vi "send.vi"() -> ()   [LabVIEW 2011]
uses:
  RabbitMQ.Client
panel:
  in  "send":bool
  in  "stop":bool
  in  "String":string="Hello world"
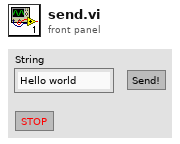
[diagram p1: front panel]
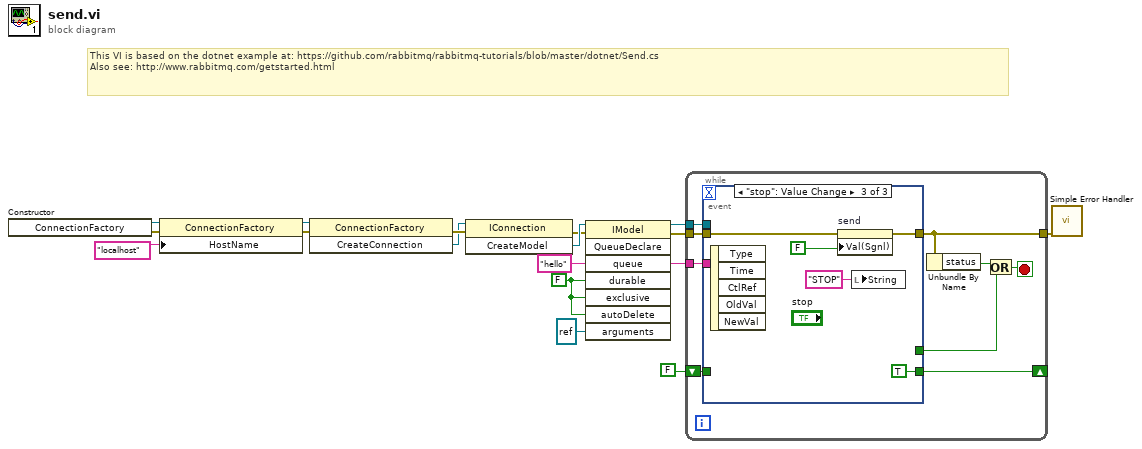
[diagram p0: block diagram]
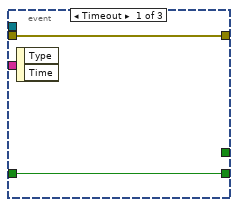
[diagram p2: hidden frame]
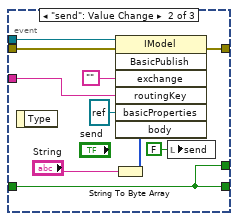
[diagram p3: hidden frame]
diagram:
  w7 = FALSE ("durable")
  w3 = "hello" ("queue")
  # "This VI is based on the dotnet example at: https://github.com/rabbitmq/rabbitmq-tutorials/blob/master/dotnet/Send.cs\nAlso see: http://www.rabbitmq.com/getstarted.html"
  n1 = constructor class="ConnectionFactory"() -> (reference out=w16:refnum<k24>, error out=w14:errorcluster)  [unwired: 3 in, 1 out]
  n2 = property class="ConnectionFactory"(reference=w16, error in=w14, "HostName"="localhost") -> (reference out=w13:refnum<k24>, error out=w12:errorcluster)
  n3 = invoke class="ConnectionFactory" method="CreateConnection"(reference=w13, error in=w12) -> (error out=w11:errorcluster, "CreateConnection"=w10:refnum<k24>)  [unwired: 1 in, 1 out]
  n4 = invoke class="IConnection" method="CreateModel"(reference=w10, error in=w11) -> (error out=w8:errorcluster, "CreateModel"=w9:refnum<k24>)  [unwired: 1 in, 1 out]
  n5 = invoke class="IModel" method="QueueDeclare"(reference=w9, error in=w8, "queue"=w3, "durable"=w7, "exclusive"=w7, "autoDelete"=w7, "arguments"=refnum<k24> refnum) -> (reference out=w5:refnum<k24>, error out=w4:errorcluster)  [unwired: 1 in, 6 out]
  n6 = while {
    tunnel: w5 -> [w25]
    tunnel: w4 -> [w24]
    tunnel: w3 -> [w23]
    tunnel: [w22] -> w2
    shift-right: [w17] -> _
    shift-left: FALSE -> [w18]
    stop <- w20 stop-if-true
    n7 = event shown="[2] \"stop\": Value Change" {
      selector: _ -> [_ _ _]
      dyn-events: _ -> [_ _ _]
      timeout: _ -> [_ _ _]
      tunnel: w25 -> [_ w37 _]
      tunnel: w24 -> [w27 w36 w41]
      tunnel: w23 -> [_ w35 _]
      tunnel: [w27 w30 w40] -> w22
      tunnel: [_ w28 _] -> w19
      tunnel: w18 -> [w26 w28 _]
      tunnel: [w26 w28 TRUE] -> w17
      event Timeout {
        n8 = event-data() -> ()  [unwired: 1 in, 2 out]
      }
      event "send": Value Change {
        n9 = event-data() -> ()  [unwired: 1 in, 1 out]
        n10 = String To Byte Array(string="String") -> (unsigned byte array=w32:u8[])
        n11 = invoke class="IModel" method="BasicPublish"(reference=w37, error in=w36, "exchange"="", "routingKey"=w35, "basicProperties"=refnum<k24> refnum, "body"=w32) -> (error out=w30:errorcluster)  [unwired: 1 in, 6 out]
        n12 = local write "send"(FALSE ("send")) -> ()
      }
      event "stop": Value Change {
        n13 = event-data() -> ()  [unwired: 1 in, 5 out]
        n14 = property on="send" class="Bool (strict)"(error in=w41, "Val(Sgnl)"=FALSE) -> (error out=w40:errorcluster)  [unwired: 1 in, 1 out]
        n15 = local write "String"("STOP" ("String")) -> ()
      }
    }
    n16 = Unbundle By Name(w22) -> ("status"=w21:bool)
    n17 = Or(x=w21, y=w19) -> (x .or. y?=w20:bool)
  }
  n18 = call <vilib>:"Simple Error Handler.vi"("error in (no error)"=w2) -> ()  [unwired: 4 in, 5 out]
